vi "InitCamera_NTSC.vi"(3 "Camera #":i32) -> (0 "error out":errorcluster={"status"=TRUE, "code"=-43, "source"=""}, 1 "QT Ref Out":T1)   [LabVIEW 2024]
doc: "This VI initializes the camera. Multiple cameras can be used and identified by altering the camera input. By changing the poly option, the user can switch between NTSC, PAL, and Advanced settings.\n\nSee the LiveFeed “behavior” in the behaviors palette for a quick sample live camera feed program."
uses:
  <userlib>/ImageProcessing/QTLIB_2595_LV86/QT_FrameGrabber.ctl
  <userlib>/ImageProcessing/CameraGlobals.vi
  <userlib>/ImageProcessing/QTLIB_2595_LV86/QT_Ref.ctl
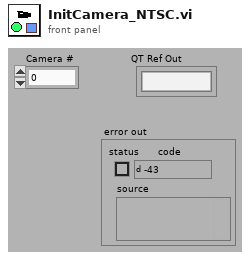
[diagram p1: front panel]
types:
  T1 = typedef "QT_Ref.ctl" = refnum<k1>
  T2 = typedef "QT_FrameGrabber.ctl" = cluster{"Name":string, "Digitizer":i32, "Input":i32, "Width":i32, "Height":i32, "Input format":enum32{"NTSC", "PAL", "Secam"}, "Frame rate":dbl, "Reserved":i32, "Dialogs":u32}
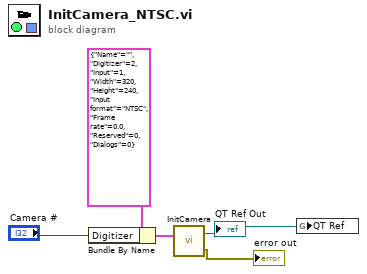
[diagram p0: block diagram]
diagram:
  n1 = Bundle By Name(cluster=T2 {"Name"="", "Digitizer"=2, "Input"=1, "Width"=320, "Height"=240, "Input format"=enum."NTSC", "Frame rate"=0.0, "Reserved"=0, "Dialogs"=0} ("Frame Grabber Settings"), "Digitizer"="Camera #") -> (w4:T2)
  n2 = call <userlib>:"InitCamera.vi"("Frame Grabber Settings"=w4) -> ("error out"=→"error out":errorcluster, "QT Ref Out"=w1:T1)  [unwired: 1 in]
  "QT Ref Out" <- w1
  n3 = global write "CameraGlobals.vi" "QT Ref"(w1) -> ()
